vi "canDataSort.vi"() -> ()   [LabVIEW 2023] (continued)
00000004    8        94\t11\t00\t55\tFF\tFF\tFF\t22\r\n      3672  1FFFFFFF   00000004    8        00\t00\tFF\tFF\tFF\tFF\tFF\tFF\r\n      3663  0CF102A7   00000004    8        30\t75\tE0\t2E\t80\tFF\tFF\tFD\r\n      3663  0CF101A7   00000004    8        68\t00\t97\tCC\t00\t19\t39\tD1\r\n      3662  1FFFFFFF   00000004    8        00\t20\tFF\tFF\tFF\tFF\tFF\tFF\r\n      3652  1FFFFFFF   00000004    8        00\t20\tFF\tFF\tFF\tFF\tFF\tFF\r\n      3649  1FFFFFFF   00000004    8        00\t00\tFF\tFF\tFF\tFF\tFF\tFF\r\n      3648  18FEF117   00000004    8        F7\t97\tCC\tCF\tFF\tFF\tFF\tFF\r\n      3648  18FB01A7   00000004    8        FF\t1F\tFF\tFF\tFF\tFF\tFF\tFF\r\n      3647  18F121F0   00000004    8        09\t33\t00\t00\tFF\tFF\tB0\t01\r\n      3646  18F108A7   00000004    8        F0\t00\t00\tFF\tFF\tFF\tFF\t45\r\n      3646  18F106A7   00000004    8        00\tF7\tFF\tFF\tFF\tFF\tFF\tB9\r\n      3682  1FFFFFFF   00000004    8        00\t20\tFF\tFF\tFF\tFF\tFF\tFF\r\n      3672  1FFFFFFF   00000004    8        00\t00\tFF\tFF\tFF\tFF\tFF\tFF\r\n      3663  0CF102A7   00000004    8        30\t75\tE0\t2E\t80\tFF\tFF\tFD\r\n      3663  0CF101A7   00000004    8        68\t00\t97\tCC\t00\t19\t39\tD1\r\n      3662  1FFFFFFF   00000004    8        00\t20\tFF\tFF\tFF\tFF\tFF\tFF\r\n      3652  1FFFFFFF   00000004    8        00\t20\tFF\tFF\tFF\tFF\tFF\tFF\r\n      3649  1FFFFFFF   00000004    8        00\t00\tFF\tFF\tFF\tFF\tFF\tFF\r\n      3648  18FEF117   00000004    8        F7\t97\tCC\tCF\tFF\tFF\tFF\tFF\r\n      3648  18FB01A7   00000004    8        FF\t1F\tFF\tFF\tFF\tFF\tFF\tFF\r\n      3647  18F121F0   00000004    8        09\t33\t00\t00\tFF\tFF\tB0\t01\r\n      3646  18F108A7   00000004    8        F0\t00\t00\tFF\tFF\tFF\tFF\t45\r\n      3683  0CF101A7   00000004    8        68\t00\t97\tCC\t00\t19\t39\tD2\r\n      3682  1FFFFFFF   00000004    8        00\t20\tFF\tFF\tFF\tFF\tFF\tFF\r\n      3672  1FFFFFFF   00000004    8        00\t00\tFF\tFF\tFF\tFF\tFF\tFF\r\n      3663  0CF102A7   00000004    8        30\t75\tE0\t2E\t80\tFF\tFF\tFD\r\n      3663  0CF101A7   00000004    8        68\t00\t97\tCC\t00\t19\t39\tD1\r\n      3662  1FFFFFFF   00000004    8        00\t20\tFF\tFF\tFF\tFF\tFF\tFF\r\n      3652  1FFFFFFF   00000004    8        00\t20\tFF\tFF\tFF\tFF\tFF\tFF\r\n      3649  1FFFFFFF   00000004    8        00\t00\tFF\tFF\tFF\tFF\tFF\tFF\r\n      3648  18FEF117   00000004    8        F7\t97\tCC\tCF\tFF\tFF\tFF\tFF\r\n      3648  18FB01A7   00000004    8        FF\t1F\tFF\tFF\tFF\tFF\tFF\tFF\r\n      3647  18F121F0   00000004    8        09\t33\t00\t00\tFF\tFF\tB0\t01\r\n      3683  0CF102A7   00000004    8        30\t75\tE0\t2E\t80\tFF\tFF\tFD\r\n      3683  0CF101A7   00000004    8        68\t00\t97\tCC\t00\t19\t39\tD2\r\n      3682  1FFFFFFF   00000004    8        00\t20\tFF\tFF\tFF\tFF\tFF\tFF\r\n      3672  1FFFFFFF   00000004    8        00\t00\tFF\tFF\tFF\tFF\tFF\tFF\r\n      3663  0CF102A7   00000004    8        30\t75\tE0\t2E\t80\tFF\tFF\tFD\r\n      3663  0CF101A7   00000004    8        68\t00\t97\tCC\t00\t19\t39\tD1\r\n      3662  1FFFFFFF   00000004    8        00\t20\tFF\tFF\tFF\tFF\tFF\tFF\r\n      3652  1FFFFFFF   00000004    8        00\t20\tFF\tFF\tFF\tFF\tFF\tFF\r\n      3649  1FFFFFFF   00000004    8        00\t00\tFF\tFF\tFF\tFF\tFF\tFF\r\n      3648  18FEF117   00000004    8        F7\t97\tCC\tCF\tFF\tFF\tFF\tFF\r\n      3648  18FB01A7   00000004    8        FF\t1F\tFF\tFF\tFF\tFF\tFF\tFF\r\n      3692  1FFFFFFF   00000004    8        00\t00\tFF\tFF\tFF\tFF\tFF\tFF\r\n      3683  0CF102A7   00000004    8        30\t75\tE0\t2E\t80\tFF\tFF\tFD\r\n      3683  0CF101A7   00000004    8        68\t00\t97\tCC\t00\t19\t39\tD2\r\n      3682  1FFFFFFF   00000004    8        00\t20\tFF\tFF\tFF\tFF\tFF\tFF\r\n      3672  1FFFFFFF   00000004    8        00\t00\tFF\tFF\tFF\tFF\tFF\tFF\r\n      3663  0CF102A7   00000004    8        30\t75\tE0\t2E\t80\tFF\tFF\tFD\r\n      3663  0CF101A7   00000004    8        68\t00\t97\tCC\t00\t19\t39\tD1\r\n      3662  1FFFFFFF   00000004    8        00\t20\tFF\tFF\tFF\tFF\tFF\tFF\r\n      3652  1FFFFFFF   00000004    8        00\t20\tFF\tFF\tFF\tFF\tFF\tFF\r\n      3649  1FFFFFFF   00000004    8        00\t00\tFF\tFF\tFF\tFF\tFF\tFF\r\n      3648  18FEF117   00000004    8        F7\t97\tCC\tCF\tFF\tFF\tFF\tFF\r\n      3693  18F106A7   00000004    8        00\tF7\tFF\tFF\tFF\tFF\tFF\tBA\r\n      3692  1FFFFFFF   00000004    8        00\t00\tFF\tFF\tFF\tFF\tFF\tFF\r\n      3683  0CF102A7   00000004    8        30\t75\tE0\t2E\t80\tFF\tFF\tFD\r\n      3683  0CF101A7   00000004    8        68\t00\t97\tCC\t00\t19\t39\tD2\r\n      3682  1FFFFFFF   00000004    8        00\t20\tFF\tFF\tFF\tFF\tFF\tFF\r\n      3672  1FFFFFFF   00000004    8        00\t00\tFF\tFF\tFF\tFF\tFF\tFF\r\n      3663  0CF102A7   00000004    8        30\t75\tE0\t2E\t80\tFF\tFF\tFD\r\n      3663  0CF101A7   00000004    8        68\t00\t97\tCC\t00\t19\t39\tD1\r\n      3662  1FFFFFFF   00000004    8        00\t20\tFF\tFF\tFF\tFF\tFF\tFF\r\n      3652  1FFFFFFF   00000004    8        00\t20\tFF\tFF\tFF\tFF\tFF\tFF\r\n      3649  1FFFFFFF   00000004    8        00\t00\tFF\tFF\tFF\tFF\tFF\tFF\r\n      3702  1FFFFFFF   00000004    8        00\t20\tFF\tFF\tFF\tFF\tFF\tFF\r\n      3693  18F106A7   00000004    8        00\tF7\tFF\tFF\tFF\tFF\tFF\tBA\r\n      3692  1FFFFFFF   00000004    8        00\t00\tFF\tFF\tFF\tFF\tFF\tFF\r\n      3683  0CF102A7   00000004    8        30\t75\tE0\t2E\t80\tFF\tFF\tFD\r\n      3683  0CF101A7   00000004    8        68\t00\t97\tCC\t00\t19\t39\tD2\r\n      3682  1FFFFFFF   00000004    8        00\t20\tFF\tFF\tFF\tFF\tFF\tFF\r\n      3672  1FFFFFFF   00000004    8        00\t00\tFF\tFF\tFF\tFF\tFF\tFF\r\n      3663  0CF102A7   00000004    8        30\t75\tE0\t2E\t80\tFF\tFF\tFD\r\n      3663  0CF101A7   00000004    8        68\t00\t97\tCC\t00\t19\t39\tD1\r\n      3662  1FFFFFFF   00000004    8        00\t20\tFF\tFF\tFF\tFF\tFF\tFF\r\n      3652  1FFFFFFF   00000004    8        00\t20\tFF\tFF\tFF\tFF\tFF\tFF\r\n      3703  0CF101A7   00000004    8        68\t00\t97\tCC\t00\t19\t39\tD3\r\n      3702  1FFFFFFF   00000004    8        00\t20\tFF\tFF\tFF\tFF\tFF\tFF\r\n      3693  18F106A7   00000004    8        00\tF7\tFF\tFF\tFF\tFF\tFF\tBA\r\n      3692  1FFFFFFF   00000004    8        00\t00\tFF\tFF\tFF\tFF\tFF\tFF\r\n      3683  0CF102A7   00000004    8        30\t75\tE0\t2E\t80\tFF\tFF\tFD\r\n      3683  0CF101A7   00000004    8        68\t00\t97\tCC\t00\t19\t39\tD2\r\n      3682  1FFFFFFF   00000004    8        00\t20\tFF\tFF\tFF\tFF\tFF\tFF\r\n      3672  1FFFFFFF   00000004    8        00\t00\tFF\tFF\tFF\tFF\tFF\tFF\r\n      3663  0CF102A7   00000004    8        30\t75\tE0\t2E\t80\tFF\tFF\tFD\r\n      3663  0CF101A7   00000004    8        68\t00\t97\tCC\t00\t19\t39\tD1\r\n      3662  1FFFFFFF   00000004    8        00\t20\tFF\tFF\tFF\tFF\tFF\tFF\r\n      3703  0CF102A7   00000004    8        30\t75\tE0\t2E\t80\tFF\tFF\tFD\r\n      3703  0CF101A7   00000004    8        68\t00\t97\tCC\t00\t19\t39\tD3\r\n      3702  1FFFFFFF   00000004    8        00\t20\tFF\tFF\tFF\tFF\tFF\tFF\r\n      3693  18F106A7   00000004    8        00\tF7\tFF\tFF\tFF\tFF\tFF\tBA\r\n      3692  1FFFFFFF   00000004    8        00\t00\tFF\tFF\tFF\tFF\tFF\tFF\r\n      3683  0CF102A7   00000004    8        30\t75\tE0\t2E\t80\tFF\tFF\tFD\r\n      3683  0CF101A7   00000004    8        68\t00\t97\tCC\t00\t19\t39\tD2\r\n      3682  1FFFFFFF   00000004    8        00\t20\tFF\tFF\tFF\tFF\tFF\tFF\r\n      3672  1FFFFFFF   00000004    8        00\t00\tFF\tFF\tFF\tFF\tFF\tFF\r\n      3663  0CF102A7   00000004    8        30\t75\tE0\t2E\t80\tFF\tFF\tFD\r\n      3663  0CF101A7   00000004    8        68\t00\t97\tCC\t00\t19\t39\tD1\r\n      3712  1FFFFFFF   00000004    8        00\t20\tFF\tFF\tFF\tFF\tFF\tFF\r\n      3703  0CF102A7   00000004    8        30\t75\tE0\t2E\t80\tFF\tFF\tFD\r\n      3703  0CF101A7   00000004    8        68\t00\t97\tCC\t00\t19\t39\tD3\r\n      3702  1FFFFFFF   00000004    8        00\t20\tFF\tFF\tFF\tFF\tFF\tFF\r\n      3693  18F106A7   00000004    8        00\tF7\tFF\tFF\tFF\tFF\tFF\tBA\r\n      3692  1FFFFFFF   00000004    8        00\t00\tFF\tFF\tFF\tFF\tFF\tFF\r\n      3683  0CF102A7   00000004    8        30\t75\tE0\t2E\t80\tFF\tFF\tFD\r\n      3683  0CF101A7   00000004    8        68\t00\t97\tCC\t00\t19\t39\tD2\r\n      3682  1FFFFFFF   00000004    8        00\t20\tFF\tFF\tFF\tFF\tFF\tFF\r\n      3672  1FFFFFFF   00000004    8        00\t00\tFF\tFF\tFF\tFF\tFF\tFF\r\n      3663  0CF102A7   00000004    8        30\t75\tE0\t2E\t80\tFF\tFF\tFD\r\n      3722  1FFFFFFF   00000004    8        00\t20\tFF\tFF\tFF\tFF\tFF\tFF\r\n      3712  1FFFFFFF   00000004    8        00\t20\tFF\tFF\tFF\tFF\tFF\tFF\r\n      3703  0CF102A7   00000004    8        30\t75\tE0\t2E\t80\tFF\tFF\tFD\r\n      3703  0CF101A7   00000004    8        68\t00\t97\tCC\t00\t19\t39\tD3\r\n      3702  1FFFFFFF   00000004    8        00\t20\tFF\tFF\tFF\tFF\tFF\tFF\r\n      3693  18F106A7   00000004    8        00\tF7\tFF\tFF\tFF\tFF\tFF\tBA\r\n      3692  1FFFFFFF   00000004    8        00\t00\tFF\tFF\tFF\tFF\tFF\tFF\r\n      3683  0CF102A7   00000004    8        30\t75\tE0\t2E\t80\tFF\tFF\tFD\r\n      3683  0CF101A7   00000004    8        68\t00\t97\tCC\t00\t19\t39\tD2\r\n      3682  1FFFFFFF   00000004    8        00\t20\tFF\tFF\tFF\tFF\tFF\tFF\r\n      3672  1FFFFFFF   00000004    8        00\t00\tFF\tFF\tFF\tFF\tFF\tFF\r\n      3723  0CF101A7   00000004    8        68\t00\t97\tCC\t00\t19\t39\tD4\r\n      3722  1FFFFFFF   00000004    8        00\t20\tFF\tFF\tFF\tFF\tFF\tFF\r\n      3712  1FFFFFFF   00000004    8        00\t20\tFF\tFF\tFF\tFF\tFF\tFF\r\n      3703  0CF102A7   00000004    8        30\t75\tE0\t2E\t80\tFF\tFF\tFD\r\n      3703  0CF101A7   00000004    8        68\t00\t97\tCC\t00\t19\t39\tD3\r\n      3702  1FFFFFFF   00000004    8        00\t20\tFF\tFF\tFF\tFF\tFF\tFF\r\n      3693  18F106A7   00000004    8        00\tF7\tFF\tFF\tFF\tFF\tFF\tBA\r\n      3692  1FFFFFFF   00000004    8        00\t00\tFF\tFF\tFF\tFF\tFF\tFF\r\n      3683  0CF102A7   00000004    8        30\t75\tE0\t2E\t80\tFF\tFF\tFD\r\n      3683  0CF101A7   00000004    8        68\t00\t97\tCC\t00\t19\t39\tD2\r\n      3682  1FFFFFFF   00000004    8        00\t20\tFF\tFF\tFF\tFF\tFF\tFF\r\n      3723  0CF102A7   00000004    8        30\t75\tE0\t2E\t80\tFF\tFF\tFD\r\n      3723  0CF101A7   00000004    8        68\t00\t97\tCC\t00\t19\t39\tD4\r\n      3722  1FFFFFFF   00000004    8        00\t20\tFF\tFF\tFF\tFF\tFF\tFF\r\n      3712  1FFFFFFF   00000004    8        00\t20\tFF\tFF\tFF\tFF\tFF\tFF\r\n      3703  0CF102A7   00000004    8        30\t75\tE0\t2E\t80\tFF\tFF\tFD\r\n      3703  0CF101A7   00000004    8        68\t00\t97\tCC\t00\t19\t39\tD3\r\n      3702  1FFFFFFF   00000004    8        00\t20\tFF\tFF\tFF\tFF\tFF\tFF\r\n      3693  18F106A7   00000004    8        00\tF7\tFF\tFF\tFF\tFF\tFF\tBA\r\n      3692  1FFFFFFF   00000004    8        00\t00\tFF\tFF\tFF\tFF\tFF\tFF\r\n      3683  0CF102A7   00000004    8        30\t75\tE0\t2E\t80\tFF\tFF\tFD\r\n      3683  0CF101A7   00000004    8        68\t00\t97\tCC\t00\t19\t39\tD2\r\n      3732  1FFFFFFF   00000004    8        00\t20\tFF\tFF\tFF\tFF\tFF\tFF\r\n      3723  0CF102A7   00000004    8        30\t75\tE0\t2E\t80\tFF\tFF\tFD\r\n      3723  0CF101A7   00000004    8        68\t00\t97\tCC\t00\t19\t39\tD4\r\n      3722  1FFFFFFF   00000004    8        00\t20\tFF\tFF\tFF\tFF\tFF\tFF\r\n      3712  1FFFFFFF   00000004    8        00\t20\tFF\tFF\tFF\tFF\tFF\tFF\r\n      3703  0CF102A7   00000004    8        30\t75\tE0\t2E\t80\tFF\tFF\tFD\r\n      3703  0CF101A7   00000004    8        68\t00\t97\tCC\t00\t19\t39\tD3\r\n      3702  1FFFFFFF   00000004    8        00\t20\tFF\tFF\tFF\tFF\tFF\tFF\r\n      3693  18F106A7   00000004    8        00\tF7\tFF\tFF\tFF\tFF\tFF\tBA\r\n      3692  1FFFFFFF   00000004    8        00\t00\tFF\tFF\tFF\tFF\tFF\tFF\r\n      3683  0CF102A7   00000004    8        30\t75\tE0\t2E\t80\tFF\tFF\tFD\r\n      3741  18F11FF0   00000004    8        FF\t3F\t90\t68\t88\t1B\t10\tDC\r\n      3732  1FFFFFFF   00000004    8        00\t20\tFF\tFF\tFF\tFF\tFF\tFF\r\n      3723  0CF102A7   00000004    8        30\t75\tE0\t2E\t80\tFF\tFF\tFD\r\n      3723  0CF101A7   00000004    8        68\t00\t97\tCC\t00\t19\t39\tD4\r\n      3722  1FFFFFFF   00000004    8        00\t20\tFF\tFF\tFF\tFF\tFF\tFF\r\n      3712  1FFFFFFF   00000004    8        00\t20\tFF\tFF\tFF\tFF\tFF\tFF\r\n      3703  0CF102A7   00000004    8        30\t75\tE0\t2E\t80\tFF\tFF\tFD\r\n      3703  0CF101A7   00000004    8        68\t00\t97\tCC\t00\t19\t39\tD3\r\n      3702  1FFFFFFF   00000004    8        00\t20\tFF\tFF\tFF\tFF\tFF\tFF\r\n      3693  18F106A7   00000004    8        00\tF7\tFF\tFF\tFF\tFF\tFF\tBA\r\n      3692  1FFFFFFF   00000004    8        00\t00\tFF\tFF\tFF\tFF\tFF\tFF\r\n      3742  18F120F0   00000004    8        2B\t75\t60\tB1\tB0\t01\tFF\tFF\r\n      3741  18F11FF0   00000004    8        FF\t3F\t90\t68\t88\t1B\t10\tDC\r\n      3732  1FFFFFFF   00000004    8        00\t20\tFF\tFF\tFF\tFF\tFF\tFF\r\n      3723  0CF102A7   00000004    8        30\t75\tE0\t2E\t80\tFF\tFF\tFD\r\n      3723  0CF101A7   00000004    8        68\t00\t97\tCC\t00\t19\t39\tD4\r\n      3722  1FFFFFFF   00000004    8        00\t20\tFF\tFF\tFF\tFF\tFF\tFF\r\n      3712  1FFFFFFF   00000004    8        00\t20\tFF\tFF\tFF\tFF\tFF\tFF\r\n      3703  0CF102A7   00000004    8        30\t75\tE0\t2E\t80\tFF\tFF\tFD\r\n      3703  0CF101A7   00000004    8        68\t00\t97\tCC\t00\t19\t39\tD3\r\n      3702  1FFFFFFF   00000004    8        00\t20\tFF\tFF\tFF\tFF\tFF\tFF\r\n      3693  18F106A7   00000004    8        00\tF7\tFF\tFF\tFF\tFF\tFF\tBA\r\n      3743  0CF101A7   00000004    8        68\t00\t97\tCC\t00\t19\t39\tD5\r\n      3742  18F120F0   00000004    8        2B\t75\t60\tB1\tB0\t01\tFF\tFF\r\n      3741  18F11FF0   00000004    8        FF\t3F\t90\t68\t88\t1B\t10\tDC\r\n      3732  1FFFFFFF   00000004    8        00\t20\tFF\tFF\tFF\tFF\tFF\tFF\r\n      3723  0CF102A7   00000004    8        30\t75\tE0\t2E\t80\tFF\tFF\tFD\r\n      3723  0CF101A7   00000004    8        68\t00\t97\tCC\t00\t19\t39\tD4\r\n      3722  1FFFFFFF   00000004    8        00\t20\tFF\tFF\tFF\tFF\tFF\tFF\r\n      3712  1FFFFFFF   00000004    8        00\t20\tFF\tFF\tFF\tFF\tFF\tFF\r\n      3703  0CF102A7   00000004    8        30\t75\tE0\t2E\t80\tFF\tFF\tFD\r\n      3703  0CF101A7   00000004    8        68\t00\t97\tCC\t00\t19\t39\tD3\r\n      3702  1FFFFFFF   00000004    8        00\t20\tFF\tFF\tFF\tFF\tFF\tFF\r\n      3743  0C3C4D4A   00000004    8        BE\tFF\tFF\t7F\t18\tFF\tFF\t5D\r\n      3743  0CF101A7   00000004    8        68\t00\t97\tCC\t00\t19\t39\tD5\r\n      3742  18F120F0   00000004    8        2B\t75\t60\tB1\tB0\t01\tFF\tFF\r\n      3741  18F11FF0   00000004    8        FF\t3F\t90\t68\t88\t1B\t10\tDC\r\n      3732  1FFFFFFF   00000004    8        00\t20\tFF\tFF\tFF\tFF\tFF\tFF\r\n      3723  0CF102A7   00000004    8        30\t75\tE0\t2E\t80\tFF\tFF\tFD\r\n      3723  0CF101A7   00000004    8        68\t00\t97\tCC\t00\t19\t39\tD4\r\n      3722  1FFFFFFF   00000004    8        00\t20\tFF\tFF\tFF\tFF\tFF\tFF\r\n      3712  1FFFFFFF   00000004    8        00\t20\tFF\tFF\tFF\tFF\tFF\tFF\r\n      3703  0CF102A7   00000004    8        30\t75\tE0\t2E\t80\tFF\tFF\tFD\r\n      3703  0CF101A7   00000004    8        68\t00\t97\tCC\t00\t19\t39\tD3\r\n      3744  0CF102A7   00000004    8        30\t75\tE0\t2E\t80\tFF\tFF\tFD\r\n      3743  0C3C4D4A   00000004    8        BE\tFF\tFF\t7F\t18\tFF\tFF\t5D\r\n      3743  0CF101A7   00000004    8        68\t00\t97\tCC\t00\t19\t39\tD5\r\n      3742  18F120F0   00000004    8        2B\t75\t60\tB1\tB0\t01\tFF\tFF\r\n      3741  18F11FF0   00000004    8        FF\t3F\t90\t68\t88\t1B\t10\tDC\r\n      3732  1FFFFFFF   00000004    8        00\t20\tFF\tFF\tFF\tFF\tFF\tFF\r\n      3723  0CF102A7   00000004    8        30\t75\tE0\t2E\t80\tFF\tFF\tFD\r\n      3723  0CF101A7   00000004    8        68\t00\t97\tCC\t00\t19\t39\tD4\r\n      3722  1FFFFFFF   00000004    8        00\t20\tFF\tFF\tFF\tFF\tFF\tFF\r\n      3712  1FFFFFFF   00000004    8        00\t20\tFF\tFF\tFF\tFF\tFF\tFF\r\n      3703  0CF102A7   00000004    8        30\t75\tE0\t2E\t80\tFF\tFF\tFD\r\n      3744  0CF103A7   00000004    8        17\t1F\t08\t60\tB1\t1F\t08\t5D\r\n      3744  0CF102A7   00000004    8        30\t75\tE0\t2E\t80\tFF\tFF\tFD\r\n      3743  0C3C4D4A   00000004    8        BE\tFF\tFF\t7F\t18\tFF\tFF\t5D\r\n      3743  0CF101A7   00000004    8        68\t00\t97\tCC\t00\t19\t39\tD5\r\n      3742  18F120F0   00000004    8        2B\t75\t60\tB1\tB0\t01\tFF\tFF\r\n      3741  18F11FF0   00000004    8        FF\t3F\t90\t68\t88\t1B\t10\tDC\r\n      3732  1FFFFFFF   00000004    8        00\t20\tFF\tFF\tFF\tFF\tFF\tFF\r\n      3723  0CF102A7   00000004    8        30\t75\tE0\t2E\t80\tFF\tFF\tFD\r\n      3723  0CF101A7   00000004    8        68\t00\t97\tCC\t00\t19\t39\tD4\r\n      3722  1FFFFFFF   00000004    8        00\t20\tFF\tFF\tFF\tFF\tFF\tFF\r\n      3712  1FFFFFFF   00000004    8        00\t20\tFF\tFF\tFF\tFF\tFF\tFF\r\n      3745  0CF104A7   00000004    8        F0\t60\t22\tFC\tFF\tFF\tFF\t5D\r\n      3744  0CF103A7   00000004    8        17\t1F\t08\t60\tB1\t1F\t08\t5D\r\n      3744  0CF102A7   00000004    8        30\t75\tE0\t2E\t80\tFF\tFF\tFD\r\n      3743  0C3C4D4A   00000004    8        BE\tFF\tFF\t7F\t18\tFF\tFF\t5D\r\n      3743  0CF101A7   00000004    8        68\t00\t97\tCC\t00\t19\t39\tD5\r\n      3742  18F120F0   00000004    8        2B\t75\t60\tB1\tB0\t01\tFF\tFF\r\n      3741  18F11FF0   00000004    8        FF\t3F\t90\t68\t88\t1B\t10\tDC\r\n      3732  1FFFFFFF   00000004    8        00\t20\tFF\tFF\tFF\tFF\tFF\tFF\r\n      3723  0CF102A7   00000004    8        30\t75\tE0\t2E\t80\tFF\tFF\tFD\r\n      3723  0CF101A7   00000004    8        68\t00\t97\tCC\t00\t19\t39\tD4\r\n      3722  1FFFFFFF   00000004    8        00\t20\tFF\tFF\tFF\tFF\tFF\tFF\r\n      3745  18F106A7   00000004    8        00\tF7\tFF\tFF\tFF\tFF\tFF\tBB\r\n      3745  0CF104A7   00000004    8        F0\t60\t22\tFC\tFF\tFF\tFF\t5D\r\n      3744  0CF103A7   00000004    8        17\t1F\t08\t60\tB1\t1F\t08\t5D\r\n      3744  0CF102A7   00000004    8        30\t75\tE0\t2E\t80\tFF\tFF\tFD\r\n      3743  0C3C4D4A   00000004    8        BE\tFF\tFF\t7F\t18\tFF\tFF\t5D\r\n      3743  0CF101A7   00000004    8        68\t00\t97\tCC\t00\t19\t39\tD5\r\n      3742  18F120F0   00000004    8        2B\t75\t60\tB1\tB0\t01\tFF\tFF\r\n      3741  18F11FF0   00000004    8        FF\t3F\t90\t68\t88\t1B\t10\tDC\r\n      3732  1FFFFFFF   00000004    8        00\t20\tFF\tFF\tFF\tFF\tFF\tFF\r\n      3723  0CF102A7   00000004    8        30\t75\tE0\t2E\t80\tFF\tFF\tFD\r\n      3723  0CF101A7   00000004    8        68\t00\t97\tCC\t00\t19\t39\tD4\r\n      3746  18F121F0   00000004    8        09\t33\t00\t00\tFF\tFF\tB0\t01\r\n      3745  18F106A7   00000004    8        00\tF7\tFF\tFF\tFF\tFF\tFF\tBB\r\n      3745  0CF104A7   00000004    8        F0\t60\t22\tFC\tFF\tFF\tFF\t5D\r\n      3744  0CF103A7   00000004    8        17\t1F\t08\t60\tB1\t1F\t08\t5D\r\n      3744  0CF102A7   00000004    8        30\t75\tE0\t2E\t80\tFF\tFF\tFD\r\n      3743  0C3C4D4A   00000004    8        BE\tFF\tFF\t7F\t18\tFF\tFF\t5D\r\n      3743  0CF101A7   00000004    8        68\t00\t97\tCC\t00\t19\t39\tD5\r\n      3742  18F120F0   00000004    8        2B\t75\t60\tB1\tB0\t01\tFF\tFF\r\n      3741  18F11FF0   00000004    8        FF\t3F\t90\t68\t88\t1B\t10\tDC\r\n      3732  1FFFFFFF   00000004    8        00\t20\tFF\tFF\tFF\tFF\tFF\tFF\r\n      3723  0CF102A7   00000004    8        30\t75\tE0\t2E\t80\tFF\tFF\tFD\r\n      3746  1FFFFFFF   00000004    8        00\t00\tFF\tFF\tFF\tFF\tFF\tFF\r\n      3746  18F121F0   00000004    8        09\t33\t00\t00\tFF\tFF\tB0\t01\r\n      3745  18F106A7   00000004    8        00\tF7\tFF\tFF\tFF\tFF\tFF\tBB\r\n      3745  0CF104A7   00000004    8        F0\t60\t22\tFC\tFF\tFF\tFF\t5D\r\n      3744  0CF103A7   00000004    8        17\t1F\t08\t60\tB1\t1F\t08\t5D\r\n      3744  0CF102A7   00000004    8        30\t75\tE0\t2E\t80\tFF\tFF\tFD\r\n      3743  0C3C4D4A   00000004    8        BE\tFF\tFF\t7F\t18\tFF\tFF\t5D\r\n      3743  0CF101A7   00000004    8        68\t00\t97\tCC\t00\t19\t39\tD5\r\n      3742  18F120F0   00000004    8        2B\t75\t60\tB1\tB0\t01\tFF\tFF\r\n      3741  18F11FF0   00000004    8        FF\t3F\t90\t68\t88\t1B\t10\tDC\r\n      3732  1FFFFFFF   00000004    8        00\t20\tFF\tFF\tFF\tFF\tFF\tFF\r\n      3752  1FFFFFFF   00000004    8        00\t00\tFF\tFF\tFF\tFF\tFF\tFF\r\n      3746  1FFFFFFF   00000004    8        00\t00\tFF\tFF\tFF\tFF\tFF\tFF\r\n      3746  18F121F0   00000004    8        09\t33\t00\t00\tFF\tFF\tB0\t01\r\n      3745  18F106A7   00000004    8        00\tF7\tFF\tFF\tFF\tFF\tFF\tBB\r\n      3745  0CF104A7   00000004    8        F0\t60\t22\tFC\tFF\tFF\tFF\t5D\r\n      3744  0CF103A7   00000004    8        17\t1F\t08\t60\tB1\t1F\t08\t5D\r\n      3744  0CF102A7   00000004    8        30\t75\tE0\t2E\t80\tFF\tFF\tFD\r\n      3743  0C3C4D4A   00000004    8        BE\tFF\tFF\t7F\t18\tFF\tFF\t5D\r\n      3743  0CF101A7   00000004    8        68\t00\t97\tCC\t00\t19\t39\tD5\r\n      3742  18F120F0   00000004    8        2B\t75\t60\tB1\tB0\t01\tFF\tFF\r\n      3741  18F11FF0   00000004    8        FF\t3F\t90\t68\t88\t1B\t10\tDC\r\n      3762  1FFFFFFF   00000004    8        00\t00\tFF\tFF\tFF\tFF\tFF\tFF\r\n      3752  1FFFFFFF   00000004    8        00\t00\tFF\tFF\tFF\tFF\tFF\tFF\r\n      3746  1FFFFFFF   00000004    8        00\t00\tFF\tFF\tFF\tFF\tFF\tFF\r\n      3746  18F121F0   00000004    8        09\t33\t00\t00\tFF\tFF\tB0\t01\r\n      3745  18F106A7   00000004    8        00\tF7\tFF\tFF\tFF\tFF\tFF\tBB\r\n      3745  0CF104A7   00000004    8        F0\t60\t22\tFC\tFF\tFF\tFF\t5D\r\n      3744  0CF103A7   00000004    8        17\t1F\t08\t60\tB1\t1F\t08\t5D\r\n      3744  0CF102A7   00000004    8        30\t75\tE0\t2E\t80\tFF\tFF\tFD\r\n      3743  0C3C4D4A   00000004    8        BE\tFF\tFF\t7F\t18\tFF\tFF\t5D\r\n      3743  0CF101A7   00000004    8        68\t00\t97\tCC\t00\t19\t39\tD5\r\n      3742  18F120F0   00000004    8        2B\t75\t60\tB1\tB0\t01\tFF\tFF\r\n      3763  0CF101A7   00000004    8        68\t00\t97\tCC\t00\t19\t39\tD6\r\n      3762  1FFFFFFF   00000004    8        00\t00\tFF\tFF\tFF\tFF\tFF\tFF\r\n      3752  1FFFFFFF   00000004    8        00\t00\tFF\tFF\tFF\tFF\tFF\tFF\r\n      3746  1FFFFFFF   00000004    8        00\t00\tFF\tFF\tFF\tFF\tFF\tFF\r\n      3746  18F121F0   00000004    8        09\t33\t00\t00\tFF\tFF\tB0\t01\r\n      3745  18F106A7   00000004    8        00\tF7\tFF\tFF\tFF\tFF\tFF\tBB\r\n      3745  0CF104A7   00000004    8        F0\t60\t22\tFC\tFF\tFF\tFF\t5D\r\n      3744  0CF103A7   00000004    8        17\t1F\t08\t60\tB1\t1F\t08\t5D\r\n      3744  0CF102A7   00000004    8        30\t75\tE0\t2E\t80\tFF\tFF\tFD\r\n      3743  0C3C4D4A   00000004    8        BE\tFF\tFF\t7F\t18\tFF\tFF\t5D\r\n      3743  0CF101A7   00000004    8        68\t00\t97\tCC\t00\t19\t39\tD5\r\n      3763  0CF102A7   00000004    8        30\t75\tE0\t2E\t80\tFF\tFF\tFD\r\n      3763  0CF101A7   00000004    8        68\t00\t97\tCC\t00\t19\t39\tD6\r\n      3762  1FFFFFFF   00000004    8        00\t00\tFF\tFF\tFF\tFF\tFF\tFF\r\n      3752  1FFFFFFF   00000004    8        00\t00\tFF\tFF\tFF\tFF\tFF\tFF\r\n      3746  1FFFFFFF   00000004    8        00\t00\tFF\tFF\tFF\tFF\tFF\tFF\r\n      3746  18F121F0   00000004    8        09\t33\t00\t00\tFF\tFF\tB0\t01\r\n      3745  18F106A7   00000004    8        00\tF7\tFF\tFF\tFF\tFF\tFF\tBB\r\n      3745  0CF104A7   00000004    8        F0\t60\t22\tFC\tFF\tFF\tFF\t5D\r\n      3744  0CF103A7   00000004    8        17\t1F\t08\t60\tB1\t1F\t08\t5D\r\n      3744  0CF102A7   00000004    8        30\t75\tE0\t2E\t80\tFF\tFF\tFD\r\n      3743  0C3C4D4A   00000004    8        BE\tFF\tFF\t7F\t18\tFF\tFF\t5D\r\n      3772  1FFFFFFF   00000004    8        00\t00\tFF\tFF\tFF\tFF\tFF\tFF\r\n      3763  0CF102A7   00000004    8        30\t75\tE0\t2E\t80\tFF\tFF\tFD\r\n      3763  0CF101A7   00000004    8        68\t00\t97\tCC\t00\t19\t39\tD6\r\n      3762  1FFFFFFF   00000004    8        00\t00\tFF\tFF\tFF\tFF\tFF\tFF\r\n      3752  1FFFFFFF   00000004    8        00\t00\tFF\tFF\tFF\tFF\tFF\tFF\r\n      3746  1FFFFFFF   00000004    8        00\t00\tFF\tFF\tFF\tFF\tFF\tFF\r\n      3746  18F121F0   00000004    8        09\t33\t00\t00\tFF\tFF\tB0\t01\r\n      3745  18F106A7   00000004    8        00\tF7\tFF\tFF\tFF\tFF\tFF\tBB\r\n      3745  0CF104A7   00000004    8        F0\t60\t22\tFC\tFF\tFF\tFF\t5D\r\n      3744  0CF103A7   00000004    8        17\t1F\t08\t60\tB1\t1F\t08\t5D\r\n      3744  0CF102A7   00000004    8        30\t75\tE0\t2E\t80\tFF\tFF\tFD\r\n      3782  1FFFFFFF   00000004    8        00\t00\tFF\tFF\tFF\tFF\tFF\tFF\r\n      3772  1FFFFFFF   00000004    8        00\t00\tFF\tFF\tFF\tFF\tFF\tFF\r\n      3763  0CF102A7   00000004    8        30\t75\tE0\t2E\t80\tFF\tFF\tFD\r\n      3763  0CF101A7   00000004    8        68\t00\t97\tCC\t00\t19\t39\tD6\r\n      3762  1FFFFFFF   00000004    8        00\t00\tFF\tFF\tFF\tFF\tFF\tFF\r\n      3752  1FFFFFFF   00000004    8        00\t00\tFF\tFF\tFF\tFF\tFF\tFF\r\n      3746  1FFFFFFF   00000004    8        00\t00\tFF\tFF\tFF\tFF\tFF\tFF\r\n      3746  18F121F0   00000004    8        09\t33\t00\t00\tFF\tFF\tB0\t01\r\n      3745  18F106A7   00000004    8        00\tF7\tFF\tFF\tFF\tFF\tFF\tBB\r\n      3745  0CF104A7   00000004    8        F0\t60\t22\tFC\tFF\tFF\tFF\t5D\r\n      3744  0CF103A7   00000004    8        17\t1F\t08\t60\tB1\t1F\t08\t5D\r\n      3783  0CF101A7   00000004    8        68\t00\t97\tCC\t00\t19\t39\tD7\r\n      3782  1FFFFFFF   00000004    8        00\t00\tFF\tFF\tFF\tFF\tFF\tFF\r\n      3772  1FFFFFFF   00000004    8        00\t00\tFF\tFF\tFF\tFF\tFF\tFF\r\n      3763  0CF102A7   00000004    8        30\t75\tE0\t2E\t80\tFF\tFF\tFD\r\n      3763  0CF101A7   00000004    8        68\t00\t97\tCC\t00\t19\t39\tD6\r\n      3762  1FFFFFFF   00000004    8        00\t00\tFF\tFF\tFF\tFF\tFF\tFF\r\n      3752  1FFFFFFF   00000004    8        00\t00\tFF\tFF\tFF\tFF\tFF\tFF\r\n      3746  1FFFFFFF   00000004    8        00\t00\tFF\tFF\tFF\tFF\tFF\tFF\r\n      3746  18F121F0   00000004    8        09\t33\t00\t00\tFF\tFF\tB0\t01\r\n      3745  18F106A7   00000004    8        00\tF7\tFF\tFF\tFF\tFF\tFF\tBB\r\n      3745  0CF104A7   00000004    8        F0\t60\t22\tFC\tFF\tFF\tFF\t5D\r\n      3783  0CF102A7   00000004    8        30\t75\tE0\t2E\t80\tFF\tFF\tFD\r\n      3783  0CF101A7   00000004    8        68\t00\t97\tCC\t00\t19\t39\tD7\r\n      3782  1FFFFFFF   00000004    8        00\t00\tFF\tFF\tFF\tFF\tFF\tFF\r\n      3772  1FFFFFFF   00000004    8        00\t00\tFF\tFF\tFF\tFF\tFF\tFF\r\n      3763  0CF102A7   00000004    8        30\t75\tE0\t2E\t80\tFF\tFF\tFD\r\n      3763  0CF101A7   00000004    8        68\t00\t97\tCC\t00\t19\t39\tD6\r\n      3762  1FFFFFFF   00000004    8        00\t00\tFF\tFF\tFF\tFF\tFF\tFF\r\n      3752  1FFFFFFF   00000004    8        00\t00\tFF\tFF\tFF\tFF\tFF\tFF\r\n      3746  1FFFFFFF   00000004    8        00\t00\tFF\tFF\tFF\tFF\tFF\tFF\r\n      3746  18F121F0   00000004    8        09\t33\t00\t00\tFF\tFF\tB0\t01\r\n      3745  18F106A7   00000004    8        00\tF7\tFF\tFF\tFF\tFF\tFF\tBB\r\n      3792  1FFFFFFF   00000004    8        00\t00\tFF\tFF\tFF\tFF\tFF\tFF\r\n      3783  0CF102A7   00000004    8        30\t75\tE0\t2E\t80\tFF\tFF\tFD\r\n      3783  0CF101A7   00000004    8        68\t00\t97\tCC\t00\t19\t39\tD7\r\n      3782  1FFFFFFF   00000004    8        00\t00\tFF\tFF\tFF\tFF\tFF\tFF\r\n      3772  1FFFFFFF   00000004    8        00\t00\tFF\tFF\tFF\tFF\tFF\tFF\r\n      3763  0CF102A7   00000004    8        30\t75\tE0\t2E\t80\tFF\tFF\tFD\r\n      3763  0CF101A7   00000004    8        68\t00\t97\tCC\t00\t19\t39\tD6\r\n      3762  1FFFFFFF   00000004    8        00\t00\tFF\tFF\tFF\tFF\tFF\tFF\r\n      3752  1FFFFFFF   00000004    8        00\t00\tFF\tFF\tFF\tFF\tFF\tFF\r\n      3746  1FFFFFFF   00000004    8        00\t00\tFF\tFF\tFF\tFF\tFF\tFF\r\n      3746  18F121F0   00000004    8        09\t33\t00\t00\tFF\tFF\tB0\t01\r\n      3793  18F106A7   00000004    8        00\tF7\tFF\tFF\tFF\tFF\tFF\tBC\r\n      3792  1FFFFFFF   00000004    8        00\t00\tFF\tFF\tFF\tFF\tFF\tFF\r\n      3783  0CF102A7   00000004    8        30\t75\tE0\t2E\t80\tFF\tFF\tFD\r\n      3783  0CF101A7   00000004    8        68\t00\t97\tCC\t00\t19\t39\tD7\r\n      3782  1FFFFFFF   00000004    8        00\t00\tFF\tFF\tFF\tFF\tFF\tFF\r\n      3772  1FFFFFFF   00000004    8        00\t00\tFF\tFF\tFF\tFF\tFF\tFF\r\n      3763  0CF102A7   00000004    8        30\t75\tE0\t2E\t80\tFF\tFF\tFD\r\n      3763  0CF101A7   00000004    8        68\t00\t97\tCC\t00\t19\t39\tD6\r\n      3762  1FFFFFFF   00000004    8        00\t00\tFF\tFF\tFF\tFF\tFF\tFF\r\n      3752  1FFFFFFF   00000004    8        00\t00\tFF\tFF\tFF\tFF\tFF\tFF\r\n      3746  1FFFFFFF   00000004    8        00\t00\tFF\tFF\tFF\tFF\tFF\tFF\r\n      3802  1FFFFFFF   00000004    8        00\t00\tFF\tFF\tFF\tFF\tFF\tFF\r\n      3793  18F106A7   00000004    8        00\tF7\tFF\tFF\tFF\tFF\tFF\tBC\r\n      3792  1FFFFFFF   00000004    8        00\t00\tFF\tFF\tFF\tFF\tFF\tFF\r\n      3783  0CF102A7   00000004    8        30\t75\tE0\t2E\t80\tFF\tFF\tFD\r\n      3783  0CF101A7   00000004    8        68\t00\t97\tCC\t00\t19\t39\tD7\r\n      3782  1FFFFFFF   00000004    8        00\t00\tFF\tFF\tFF\tFF\tFF\tFF\r\n      3772  1FFFFFFF   00000004    8        00\t00\tFF\tFF\tFF\tFF\tFF\tFF\r\n      3763  0CF102A7   00000004    8        30\t75\tE0\t2E\t80\tFF\tFF\tFD\r\n      3763  0CF101A7   00000004    8        68\t00\t97\tCC\t00\t19\t39\tD6\r\n      3762  1FFFFFFF   00000004    8        00\t00\tFF\tFF\tFF\tFF\tFF\tFF\r\n      3752  1FFFFFFF   00000004    8        00\t00\tFF\tFF\tFF\tFF\tFF\tFF\r\n      3803  0CF101A7   00000004    8        68\t00\t97\tCC\t00\t19\t39\tD8\r\n      3802  1FFFFFFF   00000004    8        00\t00\tFF\tFF\tFF\tFF\tFF\tFF\r\n      3793  18F106A7   00000004    8        00\tF7\tFF\tFF\tFF\tFF\tFF\tBC\r\n      3792  1FFFFFFF   00000004    8        00\t00\tFF\tFF\tFF\tFF\tFF\tFF\r\n      3783  0CF102A7   00000004    8        30\t75\tE0\t2E\t80\tFF\tFF\tFD\r\n      3783  0CF101A7   00000004    8        68\t00\t97\tCC\t00\t19\t39\tD7\r\n      3782  1FFFFFFF   00000004    8        00\t00\tFF\tFF\tFF\tFF\tFF\tFF\r\n      3772  1FFFFFFF   00000004    8        00\t00\tFF\tFF\tFF\tFF\tFF\tFF\r\n      3763  0CF102A7   00000004    8        30\t75\tE0\t2E\t80\tFF\tFF\tFD\r\n      3763  0CF101A7   00000004    8        68\t00\t97\tCC\t00\t19\t39\tD6\r\n      3762  1FFFFFFF   00000004    8        00\t00\tFF\tFF\tFF\tFF\tFF\tFF\r\n      3803  0CF102A7   00000004    8        30\t75\tE0\t2E\t80\tFF\tFF\tFD\r\n      3803  0CF101A7   00000004    8        68\t00\t97\tCC\t00\t19\t39\tD8\r\n      3802  1FFFFFFF   00000004    8        00\t00\tFF\tFF\tFF\tFF\tFF\tFF\r\n      3793  18F106A7   00000004    8        00\tF7\tFF\tFF\tFF\tFF\tFF\tBC\r\n      3792  1FFFFFFF   00000004    8        00\t00\tFF\tFF\tFF\tFF\tFF\tFF\r\n      3783  0CF102A7   00000004    8        30\t75\tE0\t2E\t80\tFF\tFF\tFD\r\n      3783  0CF101A7   00000004    8        68\t00\t97\tCC\t00\t19\t39\tD7\r\n      3782  1FFFFFFF   00000004    8        00\t00\tFF\tFF\tFF\tFF\tFF\tFF\r\n      3772  1FFFFFFF   00000004    8        00\t00\tFF\tFF\tFF\tFF\tFF\tFF\r\n      3763  0CF102A7   00000004    8        30\t75\tE0\t2E\t80\tFF\tFF\tFD\r\n      3763  0CF101A7   00000004    8        68\t00\t97\tCC\t00\t19\t39\tD6\r\n      3812  1FFFFFFF   00000004    8        00\t00\tFF\tFF\tFF\tFF\tFF\tFF\r\n      3803  0CF102A7   00000004    8        30\t75\tE0\t2E\t80\tFF\tFF\tFD\r\n      3803  0CF101A7   00000004    8        68\t00\t97\tCC\t00\t19\t39\tD8\r\n      3802  1FFFFFFF   00000004    8        00\t00\tFF\tFF\tFF\tFF\tFF\tFF\r\n      3793  18F106A7   00000004    8        00\tF7\tFF\tFF\tFF\tFF\tFF\tBC\r\n      3792  1FFFFFFF   00000004    8        00\t00\tFF\tFF\tFF\tFF\tFF\tFF\r\n      3783  0CF102A7   00000004    8        30\t75\tE0\t2E\t80\tFF\tFF\tFD\r\n      3783  0CF101A7   00000004    8        68\t00\t97\tCC\t00\t19\t39\tD7\r\n      3782  1FFFFFFF   00000004    8        00\t00\tFF\tFF\tFF\tFF\tFF\tFF\r\n      3772  1FFFFFFF   00000004    8        00\t00\tFF\tFF\tFF\tFF\tFF\tFF\r\n      3763  0CF102A7   00000004    8        30\t75\tE0\t2E\t80\tFF\tFF\tFD\r\n      3822  1FFFFFFF   00000004    8        00\t20\tFF\tFF\tFF\tFF\tFF\tFF\r\n      3812  1FFFFFFF   00000004    8        00\t00\tFF\tFF\tFF\tFF\tFF\tFF\r\n      3803  0CF102A7   00000004    8        30\t75\tE0\t2E\t80\tFF\tFF\tFD\r\n      3803  0CF101A7   00000004    8        68\t00\t97\tCC\t00\t19\t39\tD8\r\n      3802  1FFFFFFF   00000004    8        00\t00\tFF\tFF\tFF\tFF\tFF\tFF\r\n      3793  18F106A7   00000004    8        00\tF7\tFF\tFF\tFF\tFF\tFF\tBC\r\n      3792  1FFFFFFF   00000004    8        00\t00\tFF\tFF\tFF\tFF\tFF\tFF\r\n      3783  0CF102A7   00000004    8        30\t75\tE0\t2E\t80\tFF\tFF\tFD\r\n      3783  0CF101A7   00000004    8        68\t00\t97\tCC\t00\t19\t39\tD7\r\n      3782  1FFFFFFF   00000004    8        00\t00\tFF\tFF\tFF\tFF\tFF\tFF\r\n      3772  1FFFFFFF   00000004    8        00\t00\tFF\tFF\tFF\tFF\tFF\tFF\r\n      3823  0CF101A7   00000004    8        68\t00\t97\tCC\t00\t19\t39\tD9\r\n      3822  1FFFFFFF   00000004    8        00\t20\tFF\tFF\tFF\tFF\tFF\tFF\r\n      3812  1FFFFFFF   00000004    8        00\t00\tFF\tFF\tFF\tFF\tFF\tFF\r\n      3803  0CF102A7   00000004    8        30\t75\tE0\t2E\t80\tFF\tFF\tFD\r\n      3803  0CF101A7   00000004    8        68\t00\t97\tCC\t00\t19\t39\tD8\r\n      3802  1FFFFFFF   00000004    8        00\t00\tFF\tFF\tFF\tFF\tFF\tFF\r\n      3793  18F106A7   00000004    8        00\tF7\tFF\tFF\tFF\tFF\tFF\tBC\r\n      3792  1FFFFFFF   00000004    8        00\t00\tFF\tFF\tFF\tFF\tFF\tFF\r\n      3783  0CF102A7   00000004    8        30\t75\tE0\t2E\t80\tFF\tFF\tFD\r\n      3783  0CF101A7   00000004    8        68\t00\t97\tCC\t00\t19\t39\tD7\r\n      3782  1FFFFFFF   00000004    8        00\t00\tFF\tFF\tFF\tFF\tFF\tFF\r\n      3823  0CF102A7   00000004    8        30\t75\tE0\t2E\t80\tFF\tFF\tFD\r\n      3823  0CF101A7   00000004    8        68\t00\t97\tCC\t00\t19\t39\tD9\r\n      3822  1FFFFFFF   00000004    8        00\t20\tFF\tFF\tFF\tFF\tFF\tFF\r\n      3812  1FFFFFFF   00000004    8        00\t00\tFF\tFF\tFF\tFF\tFF\tFF\r\n      3803  0CF102A7   00000004    8        30\t75\tE0\t2E\t80\tFF\tFF\tFD\r\n      3803  0CF101A7   00000004    8        68\t00\t97\tCC\t00\t19\t39\tD8\r\n      3802  1FFFFFFF   00000004    8        00\t00\tFF\tFF\tFF\tFF\tFF\tFF\r\n      3793  18F106A7   00000004    8        00\tF7\tFF\tFF\tFF\tFF\tFF\tBC\r\n      3792  1FFFFFFF   00000004    8        00\t00\tFF\tFF\tFF\tFF\tFF\tFF\r\n      3783  0CF102A7   00000004    8        30\t75\tE0\t2E\t80\tFF\tFF\tFD\r\n      3783  0CF101A7   00000004    8        68\t00\t97\tCC\t00\t19\t39\tD7\r\n      3832  1FFFFFFF   00000004    8        00\t00\tFF\tFF\tFF\tFF\tFF\tFF\r\n      3823  0CF102A7   00000004    8        30\t75\tE0\t2E\t80\tFF\tFF\tFD\r\n      3823  0CF101A7   00000004    8        68\t00\t97\tCC\t00\t19\t39\tD9\r\n      3822  1FFFFFFF   00000004    8        00\t20\tFF\tFF\tFF\tFF\tFF\tFF\r\n      3812  1FFFFFFF   00000004    8        00\t00\tFF\tFF\tFF\tFF\tFF\tFF\r\n      3803  0CF102A7   00000004    8        30\t75\tE0\t2E\t80\tFF\tFF\tFD\r\n      3803  0CF101A7   00000004    8        68\t00\t97\tCC\t00\t19\t39\tD8\r\n      3802  1FFFFFFF   00000004    8        00\t00\tFF\tFF\tFF\tFF\tFF\tFF\r\n      3793  18F106A7   00000004    8        00\tF7\tFF\tFF\tFF\tFF\tFF\tBC\r\n      3792  1FFFFFFF   00000004    8        00\t00\tFF\tFF\tFF\tFF\tFF\tFF\r\n      3783  0CF102A7   00000004    8        30\t75\tE0\t2E\t80\tFF\tFF\tFD\r\n      3841  18F11FF0   00000004    8        FF\t3F\t90\t68\t88\t1B\t10\tEC\r\n      3832  1FFFFFFF   00000004    8        00\t00\tFF\tFF\tFF\tFF\tFF\tFF\r\n      3823  0CF102A7   00000004    8        30\t75\tE0\t2E\t80\tFF\tFF\tFD\r\n      3823  0CF101A7   00000004    8        68\t00\t97\tCC\t00\t19\t39\tD9\r\n      3822  1FFFFFFF   00000004    8        00\t20\tFF\tFF\tFF\tFF\tFF\tFF\r\n      3812  1FFFFFFF   00000004    8        00\t00\tFF\tFF\tFF\tFF\tFF\tFF\r\n      3803  0CF102A7   00000004    8        30\t75\tE0\t2E\t80\tFF\tFF\tFD\r\n      3803  0CF101A7   00000004    8        68\t00\t97\tCC\t00\t19\t39\tD8\r\n      3802  1FFFFFFF   00000004    8        00\t00\tFF\tFF\tFF\tFF\tFF\tFF\r\n      3793  18F106A7   00000004    8        00\tF7\tFF\tFF\tFF\tFF\tFF\tBC\r\n      3792  1FFFFFFF   00000004    8        00\t00\tFF\tFF\tFF\tFF\tFF\tFF\r\n      3842  18F120F0   00000004    8        2B\t75\t60\tB1\tB0\t01\tFF\tFF\r\n      3841  18F11FF0   00000004    8        FF\t3F\t90\t68\t88\t1B\t10\tEC\r\n      3832  1FFFFFFF   00000004    8        00\t00\tFF\tFF\tFF\tFF\tFF\tFF\r\n      3823  0CF102A7   00000004    8        30\t75\tE0\t2E\t80\tFF\tFF\tFD\r\n      3823  0CF101A7   00000004    8        68\t00\t97\tCC\t00\t19\t39\tD9\r\n      3822  1FFFFFFF   00000004    8        00\t20\tFF\tFF\tFF\tFF\tFF\tFF\r\n      3812  1FFFFFFF   00000004    8        00\t00\tFF\tFF\tFF\tFF\tFF\tFF\r\n      3803  0CF102A7   00000004    8        30\t75\tE0\t2E\t80\tFF\tFF\tFD\r\n      3803  0CF101A7   00000004    8        68\t00\t97\tCC\t00\t19\t39\tD8\r\n      3802  1FFFFFFF   00000004    8        00\t00\tFF\tFF\tFF\tFF\tFF\tFF\r\n      3793  18F106A7   00000004    8        00\tF7\tFF\tFF\tFF\tFF\tFF\tBC\r\n      3843  0CF101A7   00000004    8        68\t00\t97\tCC\t00\t19\t39\tDA\r\n      3842  18F120F0   00000004    8        2B\t75\t60\tB1\tB0\t01\tFF\tFF\r\n      3841  18F11FF0   00000004    8        FF\t3F\t90\t68\t88\t1B\t10\tEC\r\n      3832  1FFFFFFF   00000004    8        00\t00\tFF\tFF\tFF\tFF\tFF\tFF\r\n      3823  0CF102A7   00000004    8        30\t75\tE0\t2E\t80\tFF\tFF\tFD\r\n      3823  0CF101A7   00000004    8        68\t00\t97\tCC\t00\t19\t39\tD9\r\n      3822  1FFFFFFF   00000004    8        00\t20\tFF\tFF\tFF\tFF\tFF\tFF\r\n      3812  1FFFFFFF   00000004    8        00\t00\tFF\tFF\tFF\tFF\tFF\tFF\r\n      3803  0CF102A7   00000004    8        30\t75\tE0\t2E\t80\tFF\tFF\tFD\r\n      3803  0CF101A7   00000004    8        68\t00\t97\tCC\t00\t19\t39\tD8\r\n      3802  1FFFFFFF   00000004    8        00\t00\tFF\tFF\tFF\tFF\tFF\tFF\r\n      3843  0C3C4D4A   00000004    8        BE\tFF\tFF\t7F\t18\tFF\tFF\t5E\r\n      3843  0CF101A7   00000004    8        68\t00\t97\tCC\t00\t19\t39\tDA\r\n      3842  18F120F0   00000004    8        2B\t75\t60\tB1\tB0\t01\tFF\tFF\r\n      3841  18F11FF0   00000004    8        FF\t3F\t90\t68\t88\t1B\t10\tEC\r\n      3832  1FFFFFFF   00000004    8        00\t00\tFF\tFF\tFF\tFF\tFF\tFF\r\n      3823  0CF102A7   00000004    8        30\t75\tE0\t2E\t80\tFF\tFF\tFD\r\n      3823  0CF101A7   00000004    8        68\t00\t97\tCC\t00\t19\t39\tD9\r\n      3822  1FFFFFFF   00000004    8        00\t20\tFF\tFF\tFF\tFF\tFF\tFF\r\n      3812  1FFFFFFF   00000004    8        00\t00\tFF\tFF\tFF\tFF\tFF\tFF\r\n      3803  0CF102A7   00000004    8        30\t75\tE0\t2E\t80\tFF\tFF\tFD\r\n      3803  0CF101A7   00000004    8        68\t00\t97\tCC\t00\t19\t39\tD8\r\n      3844  0CF102A7   00000004    8        30\t75\tE0\t2E\t80\tFF\tFF\tFD\r\n      3843  0C3C4D4A   00000004    8        BE\tFF\tFF\t7F\t18\tFF\tFF\t5E\r\n      3843  0CF101A7   00000004    8        68\t00\t97\tCC\t00\t19\t39\tDA\r\n      3842  18F120F0   00000004    8        2B\t75\t60\tB1\tB0\t01\tFF\tFF\r\n      3841  18F11FF0   00000004    8        FF\t3F\t90\t68\t88\t1B\t10\tEC\r\n      3832  1FFFFFFF   00000004    8        00\t00\tFF\tFF\tFF\tFF\tFF\tFF\r\n  
